vi "pco.camera_SaveMean_Example.vi"() -> ()   [LabVIEW 2019]
uses:
  pco.camera/Camera.lvclass
  pco.recorder/Recorder.lvlib
  <vilib>/picture/picture.llb/Draw 8-Bit Pixmap.vi
  <vilib>/picture/picture.llb/Draw True-Color Pixmap.vi
panel:
  out "colormap(U8)":u32[](array[numeric])
  out "Image(U16)":u16[][](graph)
  in  "Zoom [%]":i32(c297)=26
  out "Image":picture
  out "rawImage":u16[][](array[numeric])
  in  "data_format":T1(ring)=enum."Mono16"
  in  "Image Index":u32 max=9
  in  "saveImages":bool
  in  "SavePath":path
  out "Recorded Images":u32
  in  "Quit":bool
  in  "roiY1":u64=2 min=2 max=2048 step=1
  in  "roiX1":u64=2 min=2 max=2048 step=1
  in  "roiY0":u64=1 min=1 max=2047 step=1
  in  "roiX0":u64=1 min=1 max=2047 step=1
  out "Image Height":u16
  out "Image Width":u16
  in  "dwImgCount":u32=10 caption="Required Number of Images" max=4023
  out "Error":errorcluster {"code" format="%x"}
  # "This example shows how to record an image sequence, get the mean of that sequence and save it to file afterwards.\nIt is a good starting point for writing own applications.\nBut it will not be fail save, i.e. doesnt react on errors, just handles them forward to the end\n\nUsage:\nSelect your required image count you want to average over before you start the program.\nOnce started, the camera class will be initialized and images will be recorded automatically.\nTWhen acquisition has finished the mean image is read and shown.\nNow you can crop the image using the ROI parameters and select a file path.\nBy clicking save, the mean image is saved with the selected file format using the current roi setting\nThis also finishes the program and will force an exit of the camera class"
  # "pco.labview"
  # "Camera Setup"
  # "Recording Control"
  # "Parameters for image readout"
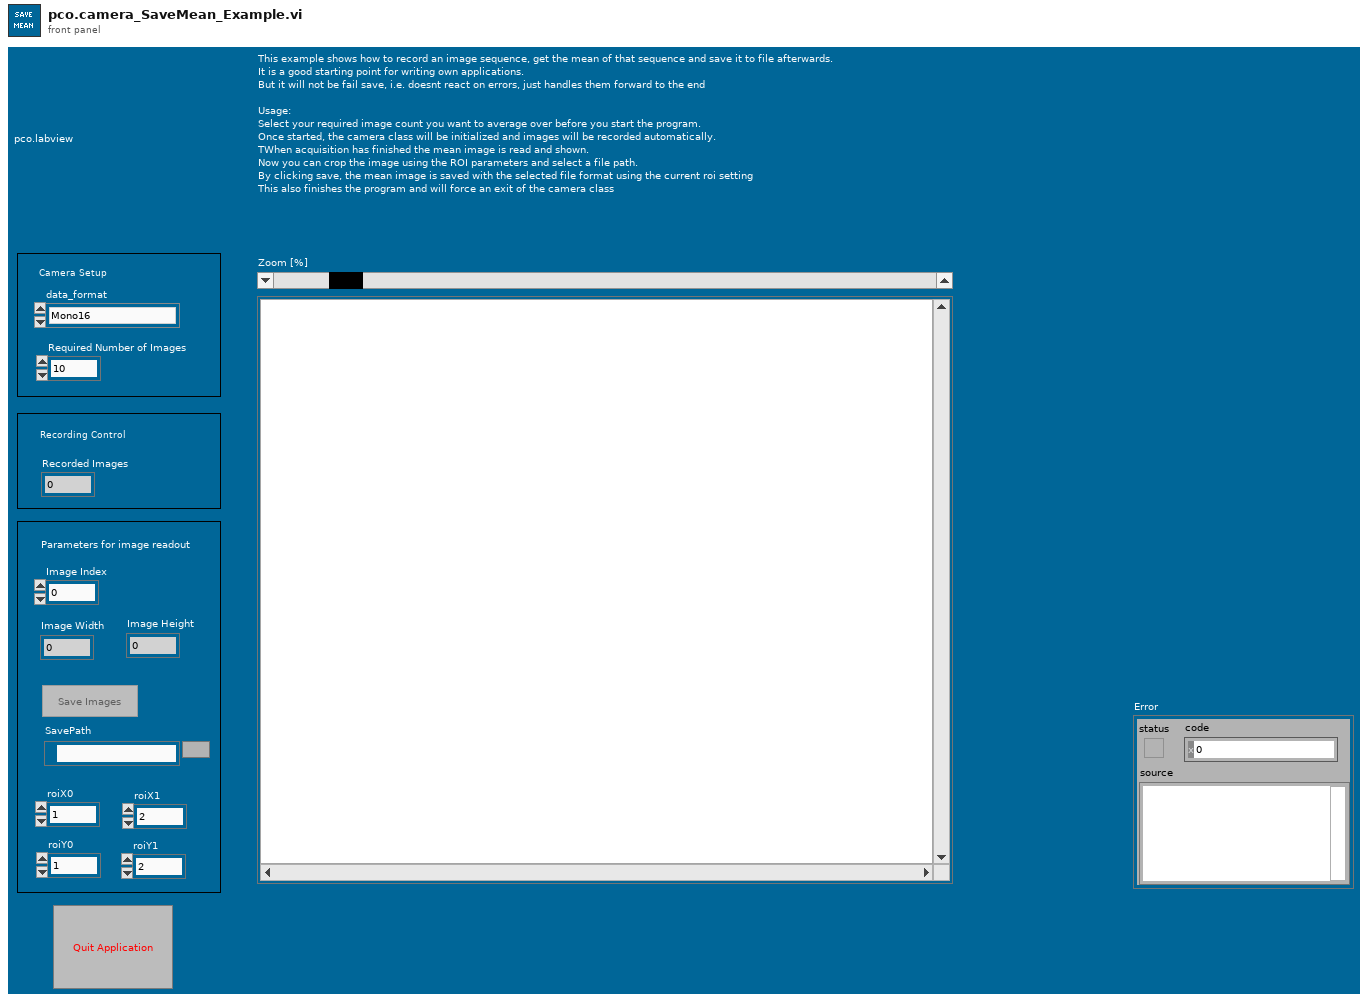
[diagram p1: front panel]
types:
  T1 = enum16{"Undefined", "Mono8", "Mono16", "BGRA8", "RGBA8", "BGRA16", "RGBA16", "CompressedMono8"}
  T2 = enum8{"Enabled", "Disabled", "Disabled and Grayed Out"}
  T3 = enum16{"sequence", "sequence non blocking", "ring buffer", "fifo", "sequence_dpcore", "sequence_non_blocking_dpcore", "ring_buffer_dpcore", "fifo_dpcore", "tif", "multitif", "pcoraw", "b16", "dicom", "multidicom"}
  T4 = typedef "Camera.lvclass/binning.ctl" = cluster{"vert":u16, "horz":u16}
  T5 = cluster{"exposure_time_s":dbl, "delay_time_s":dbl, "roi":cluster{"x0":u64, "y0":u64, "x1":u64, "y1":u64}, "timestamp_mode":u16, "pixelrate":u32, "trigger_mode":u16, "acquire_mode":u16, "metadata_mode":u16, "noisefilter_mode":u16, "binning":T4}
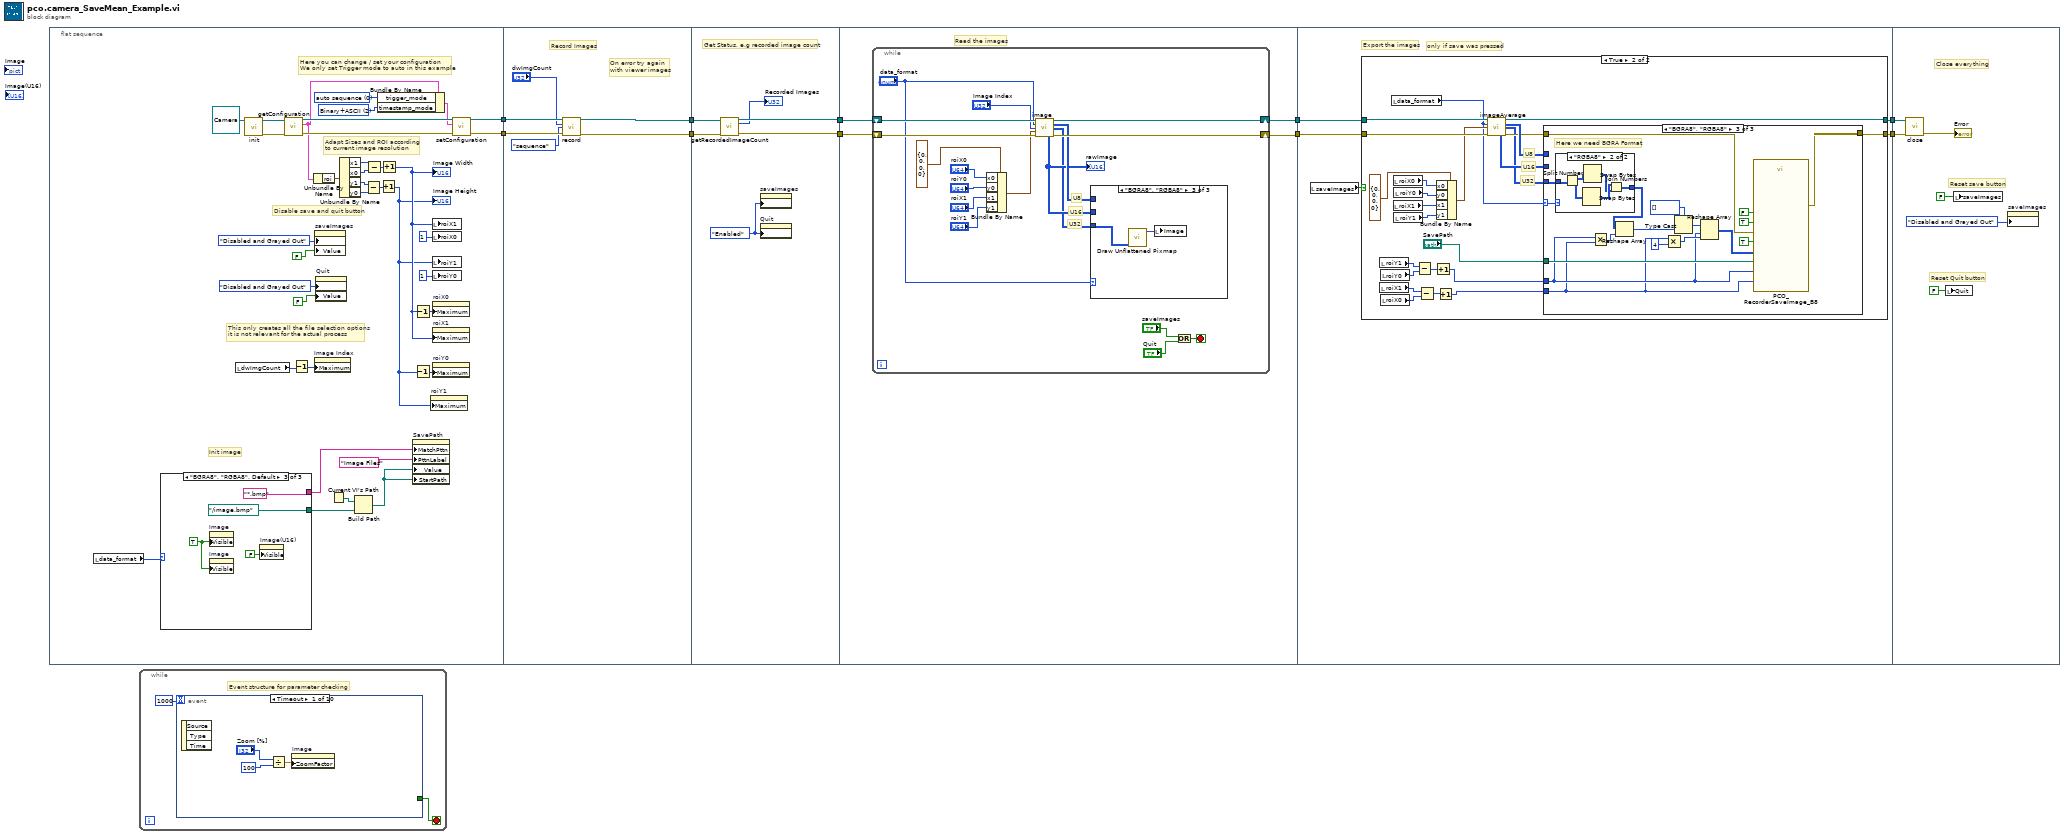
[diagram p0: block diagram]
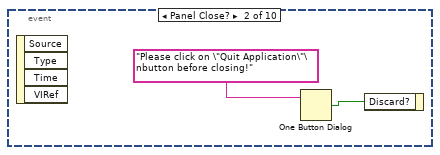
[diagram p2: hidden frame]
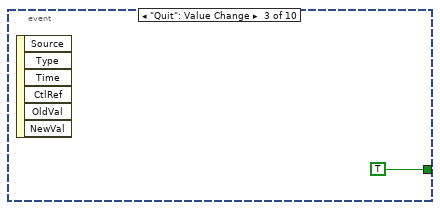
[diagram p3: hidden frame]
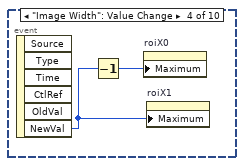
[diagram p4: hidden frame]
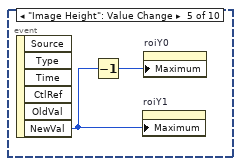
[diagram p5: hidden frame]
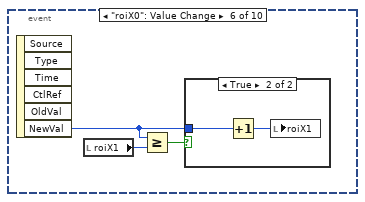
[diagram p6: hidden frame]
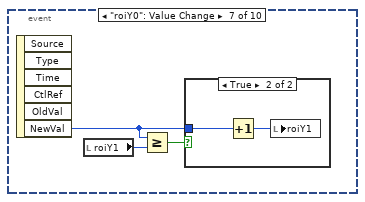
[diagram p8: hidden frame]
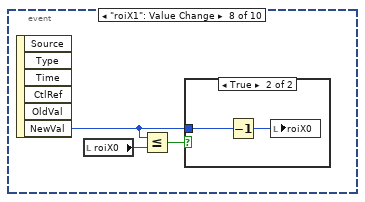
[diagram p10: hidden frame]
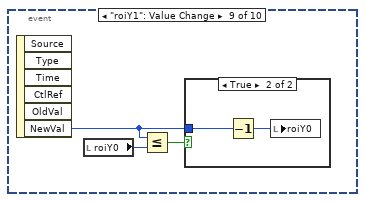
[diagram p12: hidden frame]
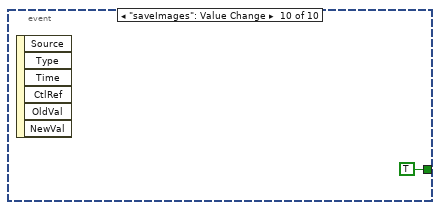
[diagram p14: hidden frame]
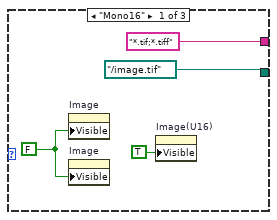
[diagram p15: hidden frame]
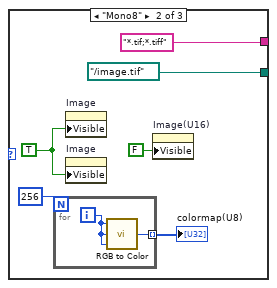
[diagram p16: hidden frame]
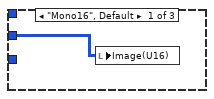
[diagram p17: hidden frame]
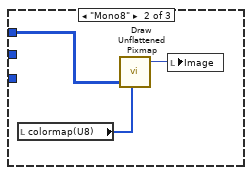
[diagram p18: hidden frame]
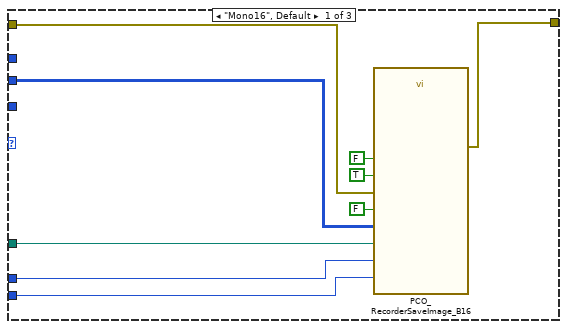
[diagram p20: hidden frame]
diagram:
  n1 = flat-sequence {
    tunnel: [w37] -> w10
    tunnel: [w36] -> w9
    tunnel: w10 -> [w68]
    tunnel: w9 -> [w67]
    tunnel: [w65] -> w8
    tunnel: [w64] -> w7
    tunnel: w8 -> [w74]
    tunnel: w7 -> [w73]
    tunnel: [w72] -> w6
    tunnel: [w71] -> w5
    tunnel: w6 -> [w77]
    tunnel: w5 -> [w78]
    tunnel: [w76] -> w4
    tunnel: [w75] -> w2
    tunnel: w4 -> [w106]
    tunnel: [w105] -> w3
    tunnel: w2 -> [w104]
    tunnel: [w103] -> w1
    tunnel: w3 -> [w182]
    tunnel: w1 -> [w181]
    frame #0 {
      w21 = u16 2 items=["OFF", "Binary", "Binary+ASCII", "ASCII"] ("TimestampMode")
      w43 = u16 0 items=["auto sequence"=0, "software trigger"=1, "external exposure start & software trigger"=2, "external exposure control"=3, "external synchronized"=4, "fast external exposure control"=5, "external CDS control"=6, "slow external exposure control"=7, "external synchronized HDSDI"=258] ("TriggerMode")
      # "Init image"
      # "This only creates all the file selection options\nit is not relevant for the actual process"
      # "Adapt Sizes and ROI according\nto current image resolution"
      # "Disable save and quit button"
      # "Here you can change / set your configuration\nWe only set Trigger mode to auto in this example"
      n2 = local read "data_format"() -> (w13:T1)
      n3 = case shown="\"BGRA8\", \"RGBA8\", Default" w13 {
        tunnel: [path "../image.tif" ("SavePath") path "../image.tif" ("SavePath") path "../image.bmp" ("SavePath")] -> w12
        tunnel: ["*.tif;*.tiff" ("pattern (all files)") "*.tif;*.tiff" ("pattern (all files)") "*.bmp" ("pattern (all files)")] -> w11
        frame "Mono16" {
          w49 = FALSE ("Visible")
          n4 = property on="Image" class="Pict"("Visible"=w49) -> ()  [unwired: 2 in, 2 out]
          n5 = property on="Image" class="Pict"("Visible"=w49) -> ()  [unwired: 2 in, 2 out]
          n6 = property on="Image(U16)" class="IntGraph (strict)"("Visible"=TRUE) -> ()  [unwired: 2 in, 2 out]
        }
        frame "Mono8" {
          w55 = TRUE ("Visible")
          n7 = for {
            N: 256 -> [_]
            tunnel: [w57] -> w54 mode=indexing
            i -> [w58]
            n8 = call <vilib>:"RGB to Color.vi"("B"=w58, "G"=w58, "R"=w58) -> ("Color"=w57:u32)
          }
          "colormap(U8)" <- w54
          n9 = property on="Image" class="Pict"("Visible"=w55) -> ()  [unwired: 2 in, 2 out]
          n10 = property on="Image" class="Pict"("Visible"=w55) -> ()  [unwired: 2 in, 2 out]
          n11 = property on="Image(U16)" class="IntGraph (strict)"("Visible"=FALSE) -> ()  [unwired: 2 in, 2 out]
        }
        frame "BGRA8", "RGBA8", Default {
          w62 = TRUE ("Visible")
          n12 = property on="Image" class="Pict"("Visible"=w62) -> ()  [unwired: 2 in, 2 out]
          n13 = property on="Image" class="Pict"("Visible"=w62) -> ()  [unwired: 2 in, 2 out]
          n14 = property on="Image(U16)" class="IntGraph (strict)"("Visible"=FALSE) -> ()  [unwired: 2 in, 2 out]
        }
      }
      n15 = local read "dwImgCount"() -> (w14:u32)
      n16 = call-dynamic "init.vi"("Camera in"=refnum<class "Camera.lvclass"> refnum ("PCOCamera in")) -> ("Camera out"=w45:refnum<class "Camera.lvclass">, "error out"=w44:errorcluster)  [unwired: 8 in]
      n17 = call-dynamic "getConfiguration.vi"("error in (no error)"=w44, "Camera in"=w45) -> ("error out"=w41:errorcluster, "configuration"=w31:T5, "Camera out"=w42:refnum<class "Camera.lvclass">)  [unwired: 7 in]
      n18 = Decrement(x=w14) -> (x-1=w15:u32)
      n19 = Unbundle By Name(w31) -> ("roi"=w30:cluster{"x0":u64, "y0":u64, "x1":u64, "y1":u64})
      n20 = property on="Image Index" class="DigNum (strict)"("Maximum"=w15) -> ()  [unwired: 2 in, 2 out]
      n21 = property on="saveImages" class="Bool (strict)"("DisabledEnum"=T2."Disabled and Grayed Out" ("Disabled"), "Value"=FALSE ("Stop")) -> ()  [unwired: 2 in, 2 out]
      n22 = property on="Quit" class="Bool (strict)"("DisabledEnum"=T2."Disabled and Grayed Out" ("Disabled"), "Value"=FALSE ("Stop")) -> ()  [unwired: 2 in, 2 out]
      n23 = Current VI's Path() -> (path=w18:path)
      n24 = Unbundle By Name(w30) -> ("x1"=w28:u64, "x0"=w29:u64, "y1"=w26:u64, "y0"=w27:u64)
      n25 = Build Path(base path=w18, name or relative path=w12) -> (appended path=w16:path)
      n26 = Subtract(x=w26, y=w27) -> (x-y=w24:u64)
      n27 = Subtract(x=w28, y=w29) -> (x-y=w25:u64)
      n28 = Bundle By Name(cluster=w31, "trigger_mode"=w43, "timestamp_mode"=w21) -> (w40:T5)
      n29 = Increment(x=w24) -> (x+1=w22:u64)
      "Image Height" <- w22
      n30 = Increment(x=w25) -> (x+1=w23:u64)
      "Image Width" <- w23
      n31 = property on="SavePath" class="Path"("MatchPttn"=w11, "PttnLabel"="Image Files" ("pattern label"), "Value"=w16, "StartPath"=w16) -> ()  [unwired: 2 in, 2 out]
      n32 = Decrement(x=w23) -> (x-1=w33:u64)
      n33 = Decrement(x=w22) -> (x-1=w32:u64)
      n34 = property on="roiY1" class="DigNum (strict)"("Maximum"=w22) -> ()  [unwired: 2 in, 2 out]
      n35 = local write "roiX1"(w23) -> ()
      n36 = local write "roiX0"(u16 1 ("roiY0")) -> ()
      n37 = local write "roiY1"(w22) -> ()
      n38 = local write "roiY0"(u16 1 ("roiY0")) -> ()
      n39 = property on="roiX0" class="DigNum (strict)"("Maximum"=w33) -> ()  [unwired: 2 in, 2 out]
      n40 = property on="roiX1" class="DigNum (strict)"("Maximum"=w23) -> ()  [unwired: 2 in, 2 out]
      n41 = property on="roiY0" class="DigNum (strict)"("Maximum"=w32) -> ()  [unwired: 2 in, 2 out]
      n42 = call-dynamic "setConfiguration.vi"("error in (no error)"=w41, "configuration"=w40, "Camera in"=w42) -> ("error out"=w36:errorcluster, "Camera out"=w37:refnum<class "Camera.lvclass">)  [unwired: 7 in]
    }
    frame #1 {
      # "On error try again \nwith viewer images"
      # "Record Images"
      n43 = call-dynamic "record.vi"("Camera in"=w68, "num_images"="dwImgCount", "record_mode"=T3."sequence", "error in (no error)"=w67) -> ("Camera out"=w65:refnum<class "Camera.lvclass">, "error out"=w64:errorcluster)  [unwired: 10 in]
    }
    frame #2 {
      w69 = T2."Enabled" ("Disabled")
      # "Get Status, e.g recorded image count"
      n44 = call-dynamic "getRecordedImageCount.vi"("Camera in"=w74, "error in (no error)"=w73) -> ("Camera out"=w72:refnum<class "Camera.lvclass">, "recorded_image_count"=→"Recorded Images":u32, "error out"=w71:errorcluster)  [unwired: 11 in]
      n45 = property on="saveImages" class="Bool (strict)"("DisabledEnum"=w69) -> ()  [unwired: 2 in, 2 out]
      n46 = property on="Quit" class="Bool (strict)"("DisabledEnum"=w69) -> ()  [unwired: 2 in, 2 out]
    }
    frame #3 {
      # "Read the images"
      n47 = while {
        shift-right: [w94] -> w76
        shift-left: w77 -> [w96]
        shift-right: [w89] -> w75
        shift-left: w78 -> [w95]
        stop <- w87 stop-if-true
        # "U32"
        # "U16"
        # "U8"
        n48 = Bundle By Name(cluster=cluster{"x0":u64, "y0":u64, "x1":u64, "y1":u64} {"x0"=0, "y0"=0, "x1"=0, "y1"=0} ("roi"), "x0"="roiX0", "y0"="roiY0", "x1"="roiX1", "y1"="roiY1") -> (w85:cluster{"x0":u64, "y0":u64, "x1":u64, "y1":u64})
        n49 = call-dynamic "image.vi"("Camera in"=w96, "data_format"="data_format", "image_index"="Image Index", "roi"=w85, "error in (no error)"=w95) -> ("Camera out"=w94:refnum<class "Camera.lvclass">, "image (U8)"=w82:u8[][], "image (U32)"=w80:u32[][], "raw_image (U16)"=w81:u16[][], "error out"=w89:errorcluster)  [unwired: 3 in, 3 out]
        "rawImage" <- w81
        n50 = case shown="\"BGRA8\", \"RGBA8\"" "data_format" {
          tunnel: w80 -> [_ _ w102]
          tunnel: w82 -> [_ w100 _]
          tunnel: w81 -> [w97 _ _]
          frame "Mono16", Default {
            n51 = local write "Image(U16)"(w97) -> ()
          }
          frame "Mono8" {
            n52 = local read "colormap(U8)"() -> (w99:u32[])
            n53 = call-poly <vilib>:"Draw Unflattened Pixmap.vi"("data"=w100, "color table"=w99) -> ("new picture"=w98:picture)  [unwired: 7 in]
            n54 = local write "Image"(w98) -> ()
          }
          frame "BGRA8", "RGBA8" {
            n55 = call-poly <vilib>:"Draw Unflattened Pixmap.vi"("data (RGB format)"=w102) -> ("new picture"=w101:picture)  [unwired: 8 in]
            n56 = local write "Image"(w101) -> ()
          }
        }
        n57 = Or(x="saveImages", y="Quit") -> (x .or. y?=w87:bool)
      }
    }
    frame #4 {
      # "only if save was pressed"
      # "Export the images"
      n58 = local read "saveImages"() -> (w107:bool)
      n59 = case shown="True" w107 {
        tunnel: w106 -> [w109 w132]
        tunnel: [w109 w123] -> w105
        tunnel: w104 -> [w108 w133]
        tunnel: [w108 w113] -> w103
        frame False {
        }
        frame True {
          # "U32"
          # "U16"
          # "U8"
          n60 = local read "roiY1"() -> (w120:u64)
          n61 = local read "roiX1"() -> (w116:u64)
          n62 = local read "roiY0"() -> (w119:u64)
          n63 = local read "roiX0"() -> (w115:u64)
          n64 = local read "data_format"() -> (w122:T1)
          n65 = local read "roiX0"() -> (w130:u64)
          n66 = local read "roiX1"() -> (w128:u64)
          n67 = local read "roiY0"() -> (w129:u64)
          n68 = local read "roiY1"() -> (w127:u64)
          n69 = Subtract(x=w120, y=w119) -> (x-y=w118:u64)
          n70 = Subtract(x=w116, y=w115) -> (x-y=w117:u64)
          n71 = Increment(x=w118) -> (x+1=w111:u64)
          n72 = Bundle By Name(cluster=cluster{"x0":u64, "y0":u64, "x1":u64, "y1":u64} {"x0"=0, "y0"=0, "x1"=0, "y1"=0} ("roi"), "x0"=w130, "y0"=w129, "x1"=w128, "y1"=w127) -> (w126:cluster{"x0":u64, "y0":u64, "x1":u64, "y1":u64})
          n73 = Increment(x=w117) -> (x+1=w112:u64)
          n74 = call-dynamic "imageAverage.vi"("Camera in"=w132, "data_format"=w122, "roi"=w126, "error in (no error)"=w133) -> ("Camera out"=w123:refnum<class "Camera.lvclass">, "image (U8)"=w125:u8[][], "image (U32)"=w110:u32[][], "raw_image (U16)"=w124:u16[][], "error out"=w114:errorcluster)  [unwired: 6 in, 1 out]
          n75 = case shown="\"BGRA8\", \"RGBA8\"" w122 {
            selector: w122 -> [_ _ w163]
            tunnel: w110 -> [_ _ w162]
            tunnel: w125 -> [_ w145 _]
            tunnel: w124 -> [w138 _ _]
            tunnel: "SavePath" -> [w136 w148 w169]
            tunnel: w112 -> [w134 w143 w152]
            tunnel: w111 -> [w135 w147 w153]
            tunnel: w114 -> [w139 w146 w167]
            tunnel: [w137 w144 w166] -> w113
            frame "Mono16", Default {
              n76 = call "PCO_RecorderSaveImage_B16.vi"("pImgBuf"=w138, "wWidth"=w134, "wHeight"=w135, "szFilePath"=w136, "error in (no error)"=w139, "isColor"=FALSE, "bIsBitmap"=FALSE, "bOverwrite"=TRUE) -> ("error out"=w137:errorcluster)  [unwired: 10 in, 1 out]
            }
            frame "Mono8" {
              n77 = call "PCO_RecorderSaveImage_B8.vi"("pImgBuf"=w145, "wWidth"=w143, "wHeight"=w147, "szFilePath"=w148, "error in (no error)"=w146, "isColor"=FALSE, "bIsBitmap"=FALSE, "bOverwrite"=TRUE) -> ("error out"=w144:errorcluster)  [unwired: 10 in, 1 out]
            }
            frame "BGRA8", "RGBA8" {
              # "Here we need BGRA Format"
              n78 = case shown="\"RGBA8\"" w163 {
                tunnel: w162 -> [w170 w176]
                tunnel: [w170 w171] -> w154
                frame Default {
                }
                frame "RGBA8" {
                  n79 = Split Number(x=w176) -> (hi(x)=w175:u16[][], lo(x)=w174:u16[][])
                  n80 = Swap Bytes(anything=w174) -> (byte swapped=w173:u16[][])
                  n81 = Swap Bytes(anything=w175) -> (byte swapped=w172:u16[][])
                  n82 = Join Numbers(hi=w173, lo=w172) -> ((hi.lo)=w171:u32[][])
                }
              }
              n83 = Multiply(x=w153, y=w152) -> (x*y=w158:u64)
              n84 = Reshape Array(w154, w158) -> (w159:u32[])
              n85 = Multiply(x=w152, y=u64 4) -> (x*y=w160:u64)
              n86 = Type Cast(type=u8[] [] ("image_list (U32)"), x=w159) -> (*(type *) &x=w161:u8[])
              n87 = Reshape Array(w161, w153, w160) -> (w155:u8[][])
              n88 = call "PCO_RecorderSaveImage_B8.vi"("pImgBuf"=w155, "wWidth"=w152, "wHeight"=w153, "szFilePath"=w169, "error in (no error)"=w167, "isColor"=TRUE, "bIsBitmap"=FALSE, "bOverwrite"=TRUE) -> ("error out"=w166:errorcluster)  [unwired: 10 in, 1 out]
            }
          }
        }
      }
    }
    frame #5 {
      # "Reset Quit button"
      # "Close everything"
      # "Reset save button"
      n89 = call-dynamic "close.vi"("error in (no error)"=w181, "Camera in"=w182) -> ("error out"=→"Error":errorcluster)  [unwired: 9 in]
      n90 = local write "Quit"(FALSE ("Stop")) -> ()
      n91 = local write "saveImages"(FALSE ("Stop")) -> ()
      n92 = property on="saveImages" class="Bool (strict)"("DisabledEnum"=T2."Disabled and Grayed Out" ("Disabled")) -> ()  [unwired: 2 in, 2 out]
    }
  }
  n93 = while {
    stop <- w183 stop-if-true
    # "Event structure for parameter checking"
    n94 = event shown="[0] Timeout" {
      selector: _ -> [_ _ _ _ _ _ _ _ _ _]
      dyn-events: _ -> [_ _ _ _ _ _ _ _ _ _]
      timeout: 1000 -> [_ _ _ _ _ _ _ _ _ _]
      tunnel: [_ _ TRUE _ _ _ _ _ _ TRUE] -> w183
      event Timeout {
        n95 = event-data() -> ()  [unwired: 1 in, 3 out]
        n96 = Divide(x="Zoom [%]", y=100 ("Zoom [%]")) -> (x/y=w187:dbl)
        n97 = property on="Image" class="Pict"("ZoomFactor"=w187) -> ()  [unwired: 2 in, 2 out]
      }
      event Panel Close? {
        n98 = event-data() -> ()  [unwired: 1 in, 4 out]
        n99 = One Button Dialog(message="Please click on \"Quit Application\"\nbutton before closing!") -> (true=w188:bool)  [unwired: 1 in]
        n100 = event-data("Discard?"=w188) -> ()  [unwired: 1 in, 1 out]
      }
      event "Quit": Value Change {
        n101 = event-data() -> ()  [unwired: 1 in, 6 out]
      }
      event "Image Width": Value Change {
        n102 = event-data() -> ("NewVal"=w191:u16)  [unwired: 1 in, 5 out]
        n103 = Decrement(x=w191) -> (x-1=w192:u16)
        n104 = property on="roiX0" class="DigNum (strict)"("Maximum"=w192) -> ()  [unwired: 2 in, 2 out]
        n105 = property on="roiX1" class="DigNum (strict)"("Maximum"=w191) -> ()  [unwired: 2 in, 2 out]
      }
      event "Image Height": Value Change {
        n106 = event-data() -> ("NewVal"=w193:u16)  [unwired: 1 in, 5 out]
        n107 = Decrement(x=w193) -> (x-1=w194:u16)
        n108 = property on="roiY1" class="DigNum (strict)"("Maximum"=w193) -> ()  [unwired: 2 in, 2 out]
        n109 = property on="roiY0" class="DigNum (strict)"("Maximum"=w194) -> ()  [unwired: 2 in, 2 out]
      }
      event "roiX0": Value Change {
        n110 = event-data() -> ("NewVal"=w195:u64)  [unwired: 1 in, 5 out]
        n111 = local read "roiX1"() -> (w197:u64)
        n112 = Greater Or Equal?(x=w195, y=w197) -> (x >= y?=w196:bool)
        n113 = case shown="True" w196 {
          tunnel: w195 -> [_ w199]
          frame False {
          }
          frame True {
            n114 = Increment(x=w199) -> (x+1=w198:u64)
            n115 = local write "roiX1"(w198) -> ()
          }
        }
      }
      event "roiY0": Value Change {
        n116 = event-data() -> ("NewVal"=w200:u64)  [unwired: 1 in, 5 out]
        n117 = local read "roiY1"() -> (w202:u64)
        n118 = Greater Or Equal?(x=w200, y=w202) -> (x >= y?=w201:bool)
        n119 = case shown="True" w201 {
          tunnel: w200 -> [_ w204]
          frame False {
          }
          frame True {
            n120 = Increment(x=w204) -> (x+1=w203:u64)
            n121 = local write "roiY1"(w203) -> ()
          }
        }
      }
      event "roiX1": Value Change {
        n122 = event-data() -> ("NewVal"=w205:u64)  [unwired: 1 in, 5 out]
        n123 = local read "roiX0"() -> (w207:u64)
        n124 = Less Or Equal?(x=w205, y=w207) -> (x <= y?=w206:bool)
        n125 = case shown="True" w206 {
          tunnel: w205 -> [_ w209]
          frame False {
          }
          frame True {
            n126 = Decrement(x=w209) -> (x-1=w208:u64)
            n127 = local write "roiX0"(w208) -> ()
          }
        }
      }
      event "roiY1": Value Change {
        n128 = event-data() -> ("NewVal"=w210:u64)  [unwired: 1 in, 5 out]
        n129 = local read "roiY0"() -> (w212:u64)
        n130 = Less Or Equal?(x=w210, y=w212) -> (x <= y?=w211:bool)
        n131 = case shown="True" w211 {
          tunnel: w210 -> [_ w214]
          frame False {
          }
          frame True {
            n132 = Decrement(x=w214) -> (x-1=w213:u64)
            n133 = local write "roiY0"(w213) -> ()
          }
        }
      }
      event "saveImages": Value Change {
        n134 = event-data() -> ()  [unwired: 1 in, 6 out]
      }
    }
  }
